vi "to wfm.vi"(11 "FFT - (RMS)":cluster{"f0":dbl, "df":dbl, "magnitude":dbl[]}[](array[cluster])) -> (3 "Array":waveform(dbl)[](array[waveform]))   [LabVIEW 2025, in "MCP Demo Application.lvlib"]
uses:
  MCP Demo Application.lvlib
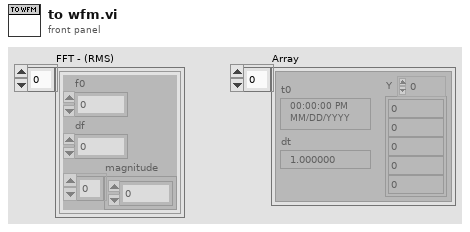
[diagram p1: front panel]
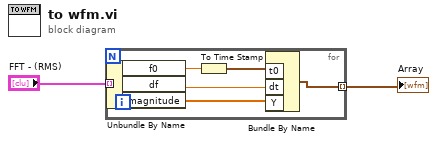
[diagram p0: block diagram]
diagram:
  n1 = for {
    tunnel: "FFT - (RMS)" -> [w8] mode=indexing
    tunnel: [w3] -> w2 mode=indexing
    n2 = Unbundle By Name(w8) -> ("f0"=w5:dbl, "df"=w6:dbl, "magnitude"=w7:dbl[])
    n3 = To Time Stamp(1:w5) -> (0:w4:timestamp)
    n4 = Bundle By Name("t0"=w4, "dt"=w6, "Y"=w7) -> (w3:waveform(dbl))  [unwired: 1 in]
  }
  "Array" <- w2
